vi "CSM - Make String Arguments Safe.vi"(2 "Argurment String":string="eaasdf->fqwvrf") -> (7 "Safe Argurment String":string)   [LabVIEW 2020, in "Communicable State Machine.lvlib"]
doc: "'->','->|','-@','-&','<-\" are key words in CSM, which should not be included in arguments. You can use this vi to make your arguments safe.\n\n<b>Inputs:</b>\n - <b>Argurment String</b>: Arguments might include '->','->|','-@','-&','<-\".\n\n<b>Outputs:</b>\n - <b>Safe Argurment String</b>: Arguments safe for CSM."
uses:
  Communicable State Machine.lvlib
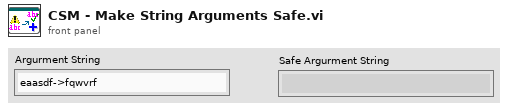
[diagram p1: front panel]
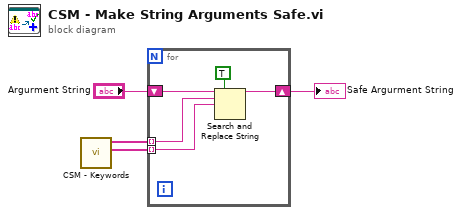
[diagram p0: block diagram]
diagram:
  n1 = call "CSM - Keywords.vi"() -> ("%[hex] Code"=w1:string[], "Source"=w2:string[])  [unwired: 10 in]
  n2 = for {
    shift-right: [w7] -> w3
    shift-left: "Argurment String" -> [w9]
    tunnel: w1 -> [w5] mode=indexing
    tunnel: w2 -> [w6] mode=indexing
    n3 = Search and Replace String(replace all?=TRUE ("replace all? (F)"), input string=w9, search string=w6, replace string=w5) -> (result string=w7:string)  [unwired: 4 in, 3 out]
  }
  "Safe Argurment String" <- w3
